vi "DangerZone(ElevatorWrist)NoCargo.vi"(3 "Wrist":T1(ring), 5 "Level":T2(ring)) -> (0 "Wrist":T1(ring), 1 "Park Horse":bool=TRUE, 2 "Level":T2(ring))   [LabVIEW 2018]
uses:
  <vilib>/Rock Robotics/WPI/ThirdParty/Phoenix-LabVIEW/Motor Controller/Get/CTRE_Phoenix_MotorController_GetSelectedSensorData.vi
panel:
  in  "Horse Upper Danger":i32=2147483647
  in  "Horse Lower Danger":i32=-5000
  in  "Intake Lower Danger":i32=105000
  in  "Intake Upper Danger":i32=300000
  in  "Elevator Lower Danger":i32=1000
  in  "Elevator Upper Danger":i32=2147483647
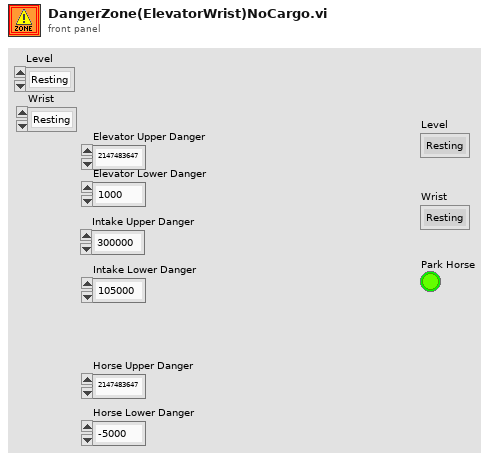
[diagram p1: front panel]
types:
  T1 = enum16{"Resting", "Hatch Ground Intake", "Hatch Place Low/Mid/CargoShip", "Hatch Place High", "Cargo Ground Intake", "Cargo Place Low/Mid", "Cargo Place High", "CargoShip Place Front", "CargoShip Place Back"}
  T2 = enum16{"Resting", "CargoShip Front", "CargoShip Back", "Cargo Mid", "Hatch Mid", "All High"}
  T3 = typedef "WPI_MotorControlDeviceRef.ctl" = cluster{"DeviceStatus":errorcluster, "Type":T4, "PWM":cluster{"PWM Channel":T5, "DeadBand":T6}, "CAN":cluster{"Device Number":u8, "SetOutput VI Ref":variant, "GetOutput VI Ref":variant, "Enable VI Ref":variant, "Disable VI Ref":variant, "Data":variant}, "Invert":bool, "DIO PWM":cluster{"PWM \"Enable\" Channel":T5, "DIOChannel":T7, "PWM Rate":dbl}}
  T4 = typedef "WPI_MotorControlType.ctl" = enum16{"PWM", "CAN", "DIO PWM"}
  T5 = typedef "FPGA_DIOPWMChannel.ctl" = enum8{"PWM 0", "PWM 1", "PWM 2", "PWM 3", "PWM 4", "PWM 5", "PWM 6", "PWM 7", "PWM 8", "PWM 9", "PWM MXP 0", "PWM MXP 1", "PWM MXP 2", "PWM MXP 3", "PWM MXP 4", "PWM MXP 5", "PWM MXP 6", "PWM MXP 7", "PWM MXP 8", "PWM MXP 9", "Invalid"}
  T6 = typedef "WPI_PWMDeadband.ctl" = cluster{"Name":string, "maxPositivePwm":i32, "minPositivePwm":i32, "centerPwm":i32, "maxNegativePwm":i32, "minNegativePwm":i32, "angularRange":u16}
  T7 = typedef "FPGA_DIOChannel.ctl" = enum8{"DIO 0", "DIO 1", "DIO 2", "DIO 3", "DIO 4", "DIO 5", "DIO 6", "DIO 7", "DIO 8", "DIO 9", "DIO MXP 0", "DIO MXP 1", "DIO MXP 2", "DIO MXP 3", "DIO MXP 4", "DIO MXP 5", "DIO MXP 6", "DIO MXP 7", "DIO MXP 8", "DIO MXP 9", "DIO MXP 10", "DIO MXP 11", "DIO MXP 12", "DIO MXP 13", "DIO MXP 14", "DIO MXP 15", "SPI Port CS1", "SPI Port CS2", "SPI Port CS3", "SPI Port MISO", "SPI Port MOSI", "Invalid"}
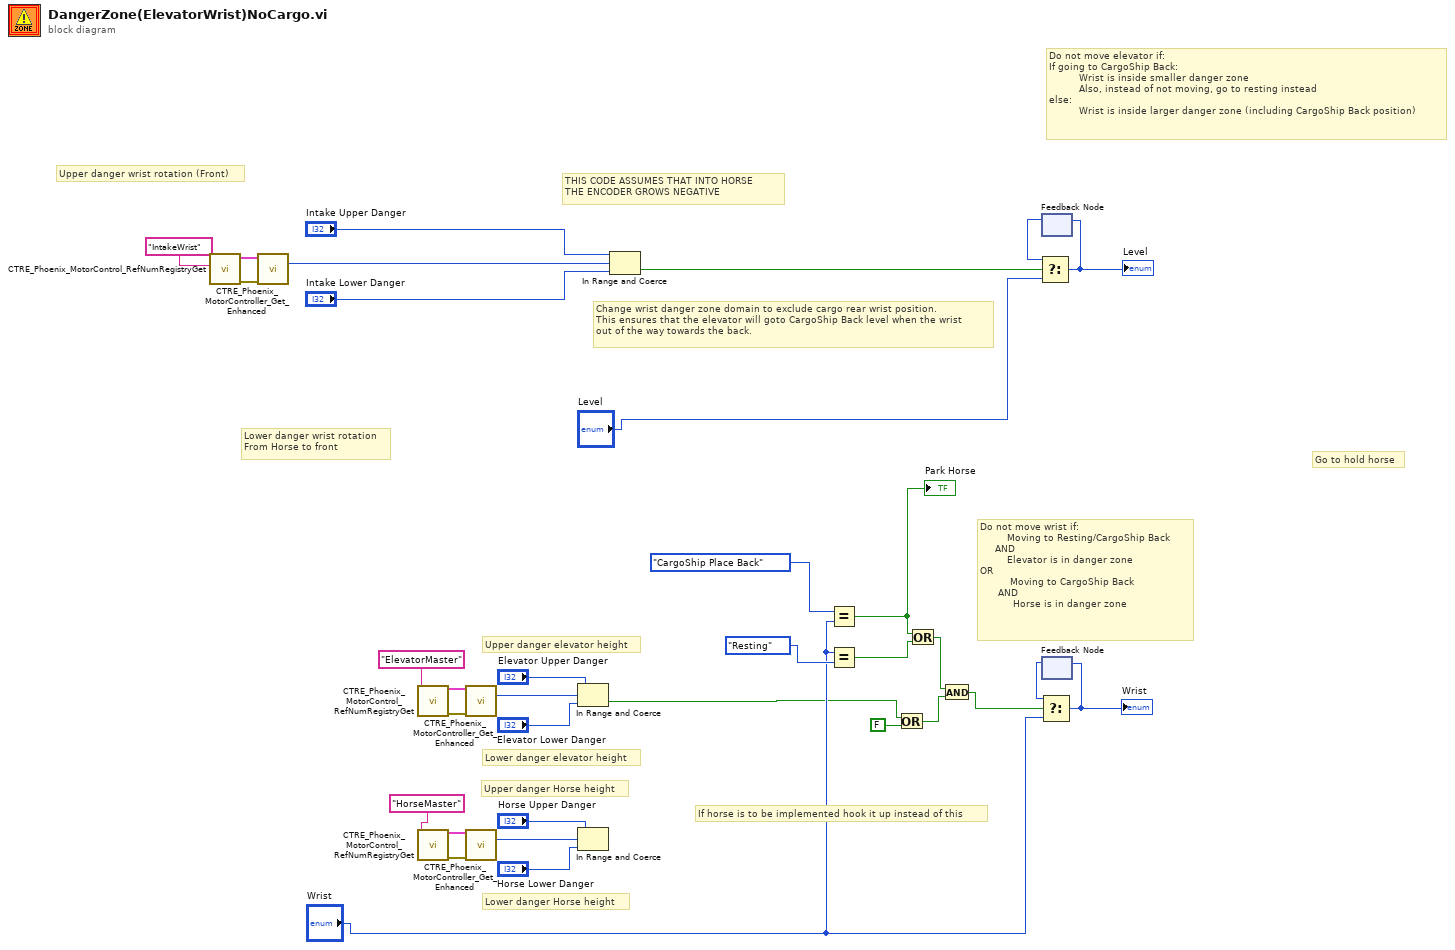
[diagram p0: block diagram]
diagram:
  # "If horse is to be implemented hook it up instead of this"
  # "Go to hold horse"
  # "Do not move elevator if:\nIf going to CargoShip Back:\n          Wrist is inside smaller danger zone\n          Also, instead of not moving, go to resting instead\nelse:\n          Wrist is inside larger danger zone (including CargoShip Back position)"
  # "Do not move wrist if:\n         Moving to Resting/CargoShip Back\n     AND\n         Elevator is in danger zone\nOR\n          Moving to CargoShip Back\n      AND\n           Horse is in danger zone"
  # "Lower danger Horse height"
  # "Upper danger Horse height"
  # "Change wrist danger zone domain to exclude cargo rear wrist position.\nThis ensures that the elevator will goto CargoShip Back level when the wrist\nout of the way towards the back."
  # "THIS CODE ASSUMES THAT INTO HORSE\nTHE ENCODER GROWS NEGATIVE"
  # "Lower danger elevator height"
  # "Upper danger wrist rotation (Front)"
  # "Lower danger wrist rotation\nFrom Horse to front"
  # "Upper danger elevator height"
  n1 = call <vilib>:"CTRE_Phoenix_MotorControl_RefNumRegistryGet.vi"("refnum name"="IntakeWrist") -> ("error out"=w33:errorcluster, "PhoenixMotorControlDevRef"=w32:T3)  [unwired: 9 in]
  n2 = call-poly <vilib>:"CTRE_Phoenix_MotorController_Get_Enhanced.vi"("PhoenixMotorControlDevRef"=w32, "error in"=w33) -> ("Position (Raw Sensor Units)"=w31:i32)  [unwired: 10 in, 3 out]
  n3 = call <vilib>:"CTRE_Phoenix_MotorControl_RefNumRegistryGet.vi"("refnum name"="ElevatorMaster") -> ("error out"=w29:errorcluster, "PhoenixMotorControlDevRef"=w28:T3)  [unwired: 9 in]
  n4 = call <vilib>:"CTRE_Phoenix_MotorControl_RefNumRegistryGet.vi"("refnum name"="HorseMaster") -> ("error out"=w16:errorcluster, "PhoenixMotorControlDevRef"=w17:T3)  [unwired: 9 in]
  n5 = call-poly <vilib>:"CTRE_Phoenix_MotorController_Get_Enhanced.vi"("PhoenixMotorControlDevRef"=w28, "error in"=w29) -> ("Position (Raw Sensor Units)"=w27:i32)  [unwired: 10 in, 3 out]
  n6 = call-poly <vilib>:"CTRE_Phoenix_MotorController_Get_Enhanced.vi"("PhoenixMotorControlDevRef"=w17, "error in"=w16) -> ("Position (Raw Sensor Units)"=w18:i32)  [unwired: 10 in, 3 out]
  n7 = In Range and Coerce(upper limit="Elevator Upper Danger", x=w27, lower limit="Elevator Lower Danger") -> (In Range?=w3:bool)  [unwired: 1 out]
  n8 = In Range and Coerce(upper limit="Horse Upper Danger", x=w18, lower limit="Horse Lower Danger") -> ()  [unwired: 2 out]
  n9 = In Range and Coerce(upper limit="Intake Upper Danger", x=w31, lower limit="Intake Lower Danger") -> (In Range?=w21:bool)  [unwired: 1 out]
  n10 = Equal?(x=T1."CargoShip Place Back" ("Wrist"), y="Wrist") -> (x = y?=w9:bool)
  "Park Horse" <- w9
  n11 = Equal?(x="Wrist", y=T1."Resting" ("Wrist")) -> (x = y?=w10:bool)
  n12 = Or(x=w3, y=FALSE) -> (x .or. y?=w4:bool)
  n13 = Or(x=w9, y=w10) -> (x .or. y?=w14:bool)
  n14 = And(x=w14, y=w4) -> (x .and. y?=w2:bool)
  n15 = feedback #1() -> (w11:T2)  [unwired: 1 in]
  n16 = Select(t=w11, s=w21, f="Level") -> (s? t:f=w24:T2)
  "Level" <- w24
  n17 = feedback-in #1(w24) -> ()
  n18 = feedback #2() -> (w22:T1)  [unwired: 1 in]
  n19 = Select(t=w22, s=w2, f="Wrist") -> (s? t:f=w23:T1)
  "Wrist" <- w23
  n20 = feedback-in #2(w23) -> ()
